vi "Main.vi"() -> ()   [LabVIEW 2017]
doc: "The myRIO Project template acquires acceleration data from the onboard accelerometer and displays the changes of acceleration values in a waveform chart."
uses:
  <vilib>/myRIO/Instrument Drivers/Onboard IO/DIO/typedefs/DIO Reference.ctl
  <vilib>/myRIO/Common/Instrument Driver Framework/Utilities/typedefs/myRIO Generic Hardware Reference.ctl
  <vilib>/myRIO/Common/Instrument Driver Framework/Utilities/typedefs/Hardware Version Enum.ctl
  <vilib>/myRIO/Common/Instrument Driver Framework/Utilities/typedefs/myRIO v1.0 Reference.ctl
  <vilib>/myRIO/Common/Instrument Driver Framework/Utilities/typedefs/Generic FPGA Reference.ctl
  <vilib>/myRIO/Common/Instrument Driver Framework/myRIO v1.0/DIO/typedefs/DIO Channels List.ctl
  <vilib>/myRIO/Common/Instrument Driver Framework/myRIO v1.0/DIO/typedefs/DIO Channels Enum.ctl
  <vilib>/userdefined/High Color/nirio_resource_hc.ctl
  <vilib>/myRIO/Instrument Drivers/Onboard Devices/Accelerometer/typedefs/Accelerometer Reference.ctl
  <vilib>/myRIO/Common/Instrument Driver Framework/myRIO v1.0/Accelerometer/typedefs/Accelerometer Channels List.ctl
  <vilib>/myRIO/Common/Instrument Driver Framework/myRIO v1.0/Accelerometer/typedefs/Accelerometer Channels Enum.ctl
  <vilib>/myRIO/Instrument Drivers/Onboard IO/AI/typedefs/AI Reference.ctl
  <vilib>/myRIO/Common/Instrument Driver Framework/myRIO v1.0/AI/typedefs/AI Channels List.ctl
  <vilib>/myRIO/Common/Instrument Driver Framework/myRIO v1.0/AI/typedefs/AI Channels Enum.ctl
  <vilib>/myRIO/Common/Instrument Driver Framework/Utilities/typedefs/Analog Scaling Constants List.ctl
  <vilib>/myRIO/Common/Instrument Driver Framework/Utilities/typedefs/Analog Scaling Constants.ctl
  <vilib>/myRIO/Common/Instrument Driver Framework/Utilities/vis/Is FPGA Ref Available.vi
  <vilib>/myRIO/Common/Instrument Driver Framework/myRIO v1.0/DIO/vis/myRIO v1.1 Open DIO.vi
  <vilib>/myRIO/Instrument Drivers/Onboard IO/DIO/vis/Write.vi
  <vilib>/myRIO/Common/Instrument Driver Framework/myRIO v1.0/AI/vis/myRIO v1.1 Open AI.vi
  <vilib>/myRIO/Instrument Drivers/Onboard IO/AI/vis/Read.vi
  <vilib>/myRIO/Instrument Drivers/Onboard IO/DIO/vis/Read.vi
  <vilib>/myRIO/Common/Instrument Driver Framework/myRIO v1.0/Accelerometer/vis/myRIO v1.1 Open Accelerometer.vi
  <vilib>/myRIO/Instrument Drivers/Onboard Devices/Accelerometer/vis/Read.vi
  <vilib>/myRIO/Common/Instrument Driver Framework/Utilities/vis/Validate Channels.vi
  <vilib>/myRIO/Common/Instrument Driver Framework/myRIO v1.0/DIO/vis/myRIO v1.0 Reserve DIO.vi
  <vilib>/myRIO/Common/Instrument Driver Framework/myRIO v1.0/AI/vis/myRIO v1.0 Reserve AI.vi
  <vilib>/myRIO/Common/Instrument Driver Framework/myRIO v1.0/Accelerometer/vis/myRIO v1.0 Reserve Accelerometer.vi
  <vilib>/myRIO/Common/Instrument Driver Framework/myRIO v1.0/UART/vis/myRIO v1.0 Close UART.vi
  <vilib>/myRIO/Common/Instrument Driver Framework/myRIO v1.0/Resource Manager/vis/myRIO v1.0 Reserve Channel List.vi
  <vilib>/myRIO/Common/Instrument Driver Framework/myRIO v1.0/DIO/vis/myRIO v1.0 Build MUX Configuration DIO.vi
  <vilib>/myRIO/Common/Instrument Driver Framework/myRIO v1.0/AI/vis/myRIO v1.0 Build MUX Configuration AI.vi
  <vilib>/myRIO/Common/Instrument Driver Framework/myRIO v1.0/Accelerometer/vis/myRIO v1.0 Build MUX Configuration Accelerometer.vi
  <vilib>/myRIO/Common/Instrument Driver Framework/myRIO v1.0/Resource Manager/vis/myRIO v1.0 Reserve Channel.vi
  <vilib>/myRIO/Common/Instrument Driver Framework/myRIO v1.0/Resource Manager/vis/myRIO v1.0 Unreserve Channel.vi
  <vilib>/myRIO/Common/Instrument Driver Framework/myRIO v1.0/Resource Manager/vis/myRIO v1.0 Create Configuration List.vi
  <vilib>/myRIO/Common/Instrument Driver Framework/myRIO v1.0/Resource Manager/vis/myRIO v1.0 Build Mutex Name.vi
  globals.vi
  <vilib>/Utility/VariantDataType/GetNumericInfo.vi
  <vilib>/Utility/error.llb/Error Cluster From Error Code.vi
  <vilib>/myRIO/Common/Instrument Driver Framework/myRIO v1.0/myRIO v1.1 Open.vi
  <vilib>/myRIO/Common/Instrument Driver Framework/myRIO v1.0/Accelerometer/vis/myRIO v1.0 Get Scaling Constant Accelerometer.vi
  <vilib>/myRIO/Common/Instrument Driver Framework/Utilities/vis/IO Manager.vi
  <vilib>/myRIO/Common/Instrument Driver Framework/Utilities/vis/Configuration Manager.vi
  <vilib>/myRIO/Common/Instrument Driver Framework/myRIO v1.0/myRIO v1.0 Close.vi
  <vilib>/myRIO/Common/Instrument Driver Framework/myRIO v1.0/Accelerometer/vis/myRIO v1.0 Read Accelerometer.vi
  <vilib>/myRIO/Common/Instrument Driver Framework/myRIO v1.0/Resource Manager/vis/myRIO v1.0 Configure IO.vi
  <vilib>/myRIO/Common/Instrument Driver Framework/myRIO v1.0/DIO/vis/myRIO v1.0 Read DIO.vi
  <vilib>/myRIO/Common/Instrument Driver Framework/myRIO v1.0/AI/vis/myRIO v1.0 Get Scaling Constants AI.vi
  <vilib>/myRIO/Common/Instrument Driver Framework/myRIO v1.0/AI/vis/myRIO v1.0 Read AI.vi
  <vilib>/myRIO/Common/Instrument Driver Framework/myRIO v1.0/DIO/vis/myRIO v1.0 Write DIO.vi
  <vilib>/myRIO/Common/Instrument Driver Framework/Utilities/vis/FPGA Ref Manager.vi
  <vilib>/myRIO/Common/Instrument Driver Framework/myRIO v1.0/myRIO v1.0 Reset FPGA.vi
  <vilib>/myRIO/Common/Instrument Driver Framework/myRIO v1.0/IRQ/vis/myRIO v1.0 IRQ Info FGV.vi
  <vilib>/myRIO/Common/Instrument Driver Framework/myRIO v1.0/IRQ/vis/myRIO v1.0 Timer IRQ Info FGV.vi
  <vilib>/myRIO/Common/Instrument Driver Framework/myRIO v1.0/IRQ/vis/myRIO v1.0 ISR Agent.vi
  <vilib>/myRIO/Express VI/Onboard Devices/Accelerometer/Accelerometer Express VI.xnode
  <vilib>/myRIO/Instrument Drivers/Onboard Devices/Accelerometer/vis/myRIO Accelerometer Open.xnode
  <vilib>/myRIO/Express VI/Onboard Devices/Button/Button Express VI.xnode
  <vilib>/myRIO/Instrument Drivers/Onboard IO/DIO/vis/myRIO DIO Open.xnode
  <vilib>/myRIO/Express VI/Onboard IO/AI/AI Express VI.xnode
  <vilib>/myRIO/Instrument Drivers/Onboard IO/AI/vis/myRIO AI Open.xnode
  <vilib>/myRIO/Express VI/Onboard Devices/LED/LED Express VI.xnode
  <vilib>/myRIO/Instrument Drivers/Utilities/Utilities.lvlib
  <vilib>/myRIO/Instrument Drivers/Onboard IO/AI/AI.lvlib
  <vilib>/myRIO/Instrument Drivers/Onboard IO/DIO/DIO.lvlib
  <vilib>/myRIO/Instrument Drivers/Onboard Devices/Accelerometer/Accelerometer.lvlib
panel:
  out "theft text":string
  out "Anti-Theft System Active":bool
  out "Local Request From Main":bool
  out "flag4":bool
  out "flag3":bool
  out "flag2":bool
  out "flag1":bool
  out "Count Down":dbl
  out "distance":dbl
  in  "setPos":bool
  out "y":dbl
  out "z":dbl
  out "x":dbl
  in  "correctPass":bool
  out "Main Controller Status":string
  out "String 2":string
  in  "Button":bool
  out "Slide 2":u8(slide) scale=0.0..100.0
  out "String":string
  out "Status":dbl
  out "buff":dbl
  in  "Main Controller IP":string
  out "Thermometer 2":dbl(slide) scale=10.0..35.0
  out "temp":dbl
  out "Slide":u8(slide) scale=0.0..100.0
  # "- If the local controller is disconected from the main controller, local cooling (Arming) is activated\n\n- Local Controller and Main controller start in the local state.\n\n- To terminate local control, hold the local controller button on the MyRio Device. A password will be sent to main controller.\n\n- To enter local cooling manually, hold the local controller button after a request has been given by the main controller to enter local cooling.\n\n- On the main controller, hold down the \"Enable Local Cooling\" Button to toggle the state. When  the state is true, the local controller button can be pressed to activate local cooling"
  # "- When the Anti-Theft system is active, moving the device will trigger the Detonation sequence. 2 different thresholds can be set in the block diagram. The distance of the movement, and the duration of the movement. The duration is there to prevent the  device being triggered by quick vibrations.\n\n- After being triggered, it will countdown from 60 seconds. This can only be deactivated from the main controller with a password.\n\n- After detonation, it will be stuck in an Inert state and can no longer be used."
  # "Statuses\n\n0 - Waiting\n1 - Main Cooling\n2 - Local Cooling\n3 - Detonation\n4 - Detonated"
  # "Detonation Alert"
  # "Nuclear Rod"
  # "Both Need to be activated to Start Local Control"
  # "Local Controller Button"
  # "The local controller and main controller will always attempt to connect to eachother when possible. Make sure the IPs at both ends are correct."
  # "(Hold For 2 Seconds)"
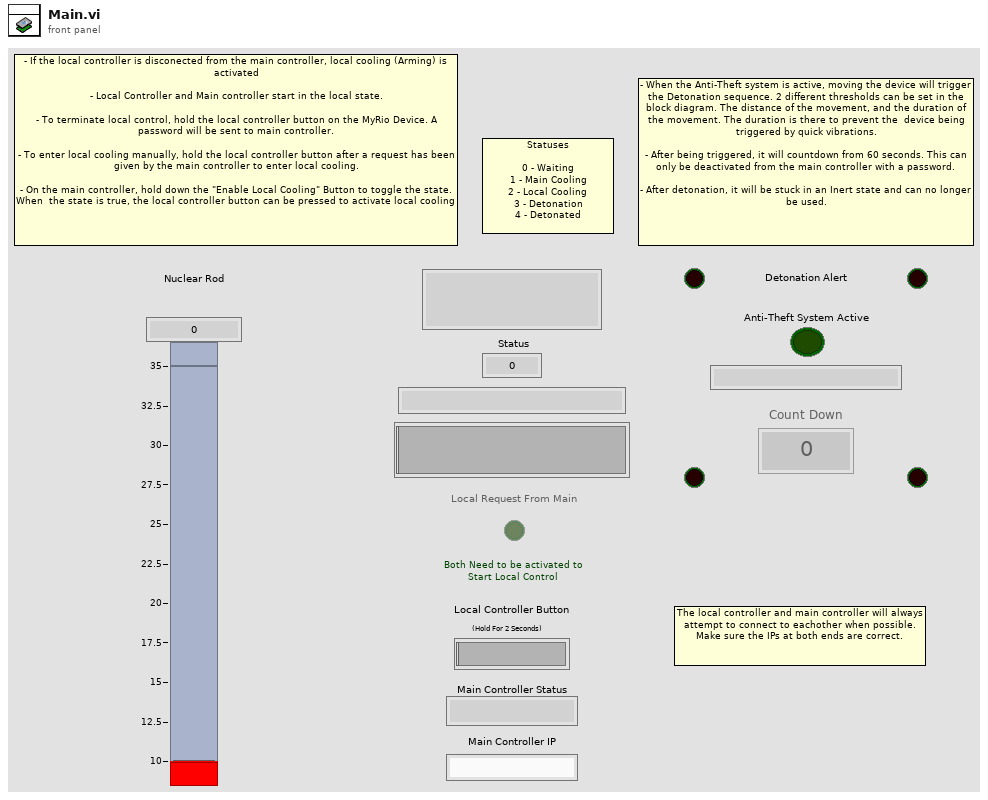
[diagram p1: front panel]
types:
  T1 = typedef "DIO.lvlib/DIO Reference.ctl" = cluster{"myRIO Reference":T2, "DIO Channels List":T6}
  T2 = typedef "myRIO Generic Hardware Reference.ctl" = cluster{"myRIO Model":T3, "myRIO Hardware Reference":T4}
  T3 = typedef "Hardware Version Enum.ctl" = enum16{"Unknown", "myRIO-1900", "myRIO-1950", "roboRIO", "NI ELVIS RIO CM"}
  T4 = typedef "myRIO v1.0 Reference.ctl" = cluster{"Generic FPGA Reference":T5, "Allow multiple opens":bool}
  T5 = typedef "Generic FPGA Reference.ctl" = refnum<k20>
  T6 = typedef "DIO Channels List.ctl" = T7[]
  T7 = typedef "DIO Channels Enum.ctl" = enum16{"Not Connected", "C/DIO0", "C/DIO1", "C/DIO2", "C/DIO3", "C/DIO4", "C/DIO5", "C/DIO6", "C/DIO7", "A/DIO0", "A/DIO1", "A/DIO2", "A/DIO3", "A/DIO4", "A/DIO5", "A/DIO6", "A/DIO7", "A/DIO8", "A/DIO9", "A/DIO10", "A/DIO11", "A/DIO12", "A/DIO13", "A/DIO14", "A/DIO15", "B/DIO0", "B/DIO1", "B/DIO2", "B/DIO3", "B/DIO4", "B/DIO5", "B/DIO6", "B/DIO7", "B/DIO8", "B/DIO9", "B/DIO10", "B/DIO11", "B/DIO12", "B/DIO13", "B/DIO14", "B/DIO15", "LED0", "LED1", "LED2", "LED3", "Button0", "DIO/DIO0", "DIO/DIO1", "DIO/DIO2", "DIO/DIO3", "DIO/DIO4", "DIO/DIO5", "DIO/DIO6", "DIO/DIO7", "DIO/DIO8", "DIO/DIO9", "SPI/CS0", "SPI/CS1", "SPI/CS2", "SPI/CS3", "LED RADIO (Green)", "LED RADIO (Red)", "LED COMM (Green)", "LED COMM (Red)", "LED MODE (Green)", "LED MODE (Red)"}
  T8 = typedef "nirio_resource_hc.ctl" = tag
  T9 = typedef "Accelerometer.lvlib/Accelerometer Reference.ctl" = cluster{"myRIO Reference":T2, "Accelerometer Channels List":T10, "LSB Weight":dbl}
  T10 = typedef "Accelerometer Channels List.ctl" = T11[]
  T11 = typedef "Accelerometer Channels Enum.ctl" = enum16{"Not Connected", "X-Axis", "Y-Axis", "Z-Axis"}
  T12 = typedef "AI.lvlib/AI Reference.ctl" = cluster{"myRIO Reference":T2, "AI Channels List":T13, "AI Scaling Constants List":T15}
  T13 = typedef "AI Channels List.ctl" = T14[]
  T14 = typedef "AI Channels Enum.ctl" = enum16{"Not Connected", "AudioIn/Left", "AudioIn/Right", "C/AI0", "C/AI1", "A/AI0", "A/AI1", "A/AI2", "A/AI3", "B/AI0", "B/AI1", "B/AI2", "B/AI3", "AI/AI0", "AI/AI1", "AI/AI2", "AI/AI3"}
  T15 = typedef "Analog Scaling Constants List.ctl" = T16[]
  T16 = typedef "Analog Scaling Constants.ctl" = cluster{"LSB Weight (Volts)":dbl, "Offset (Volts)":dbl, "Signed?":bool}
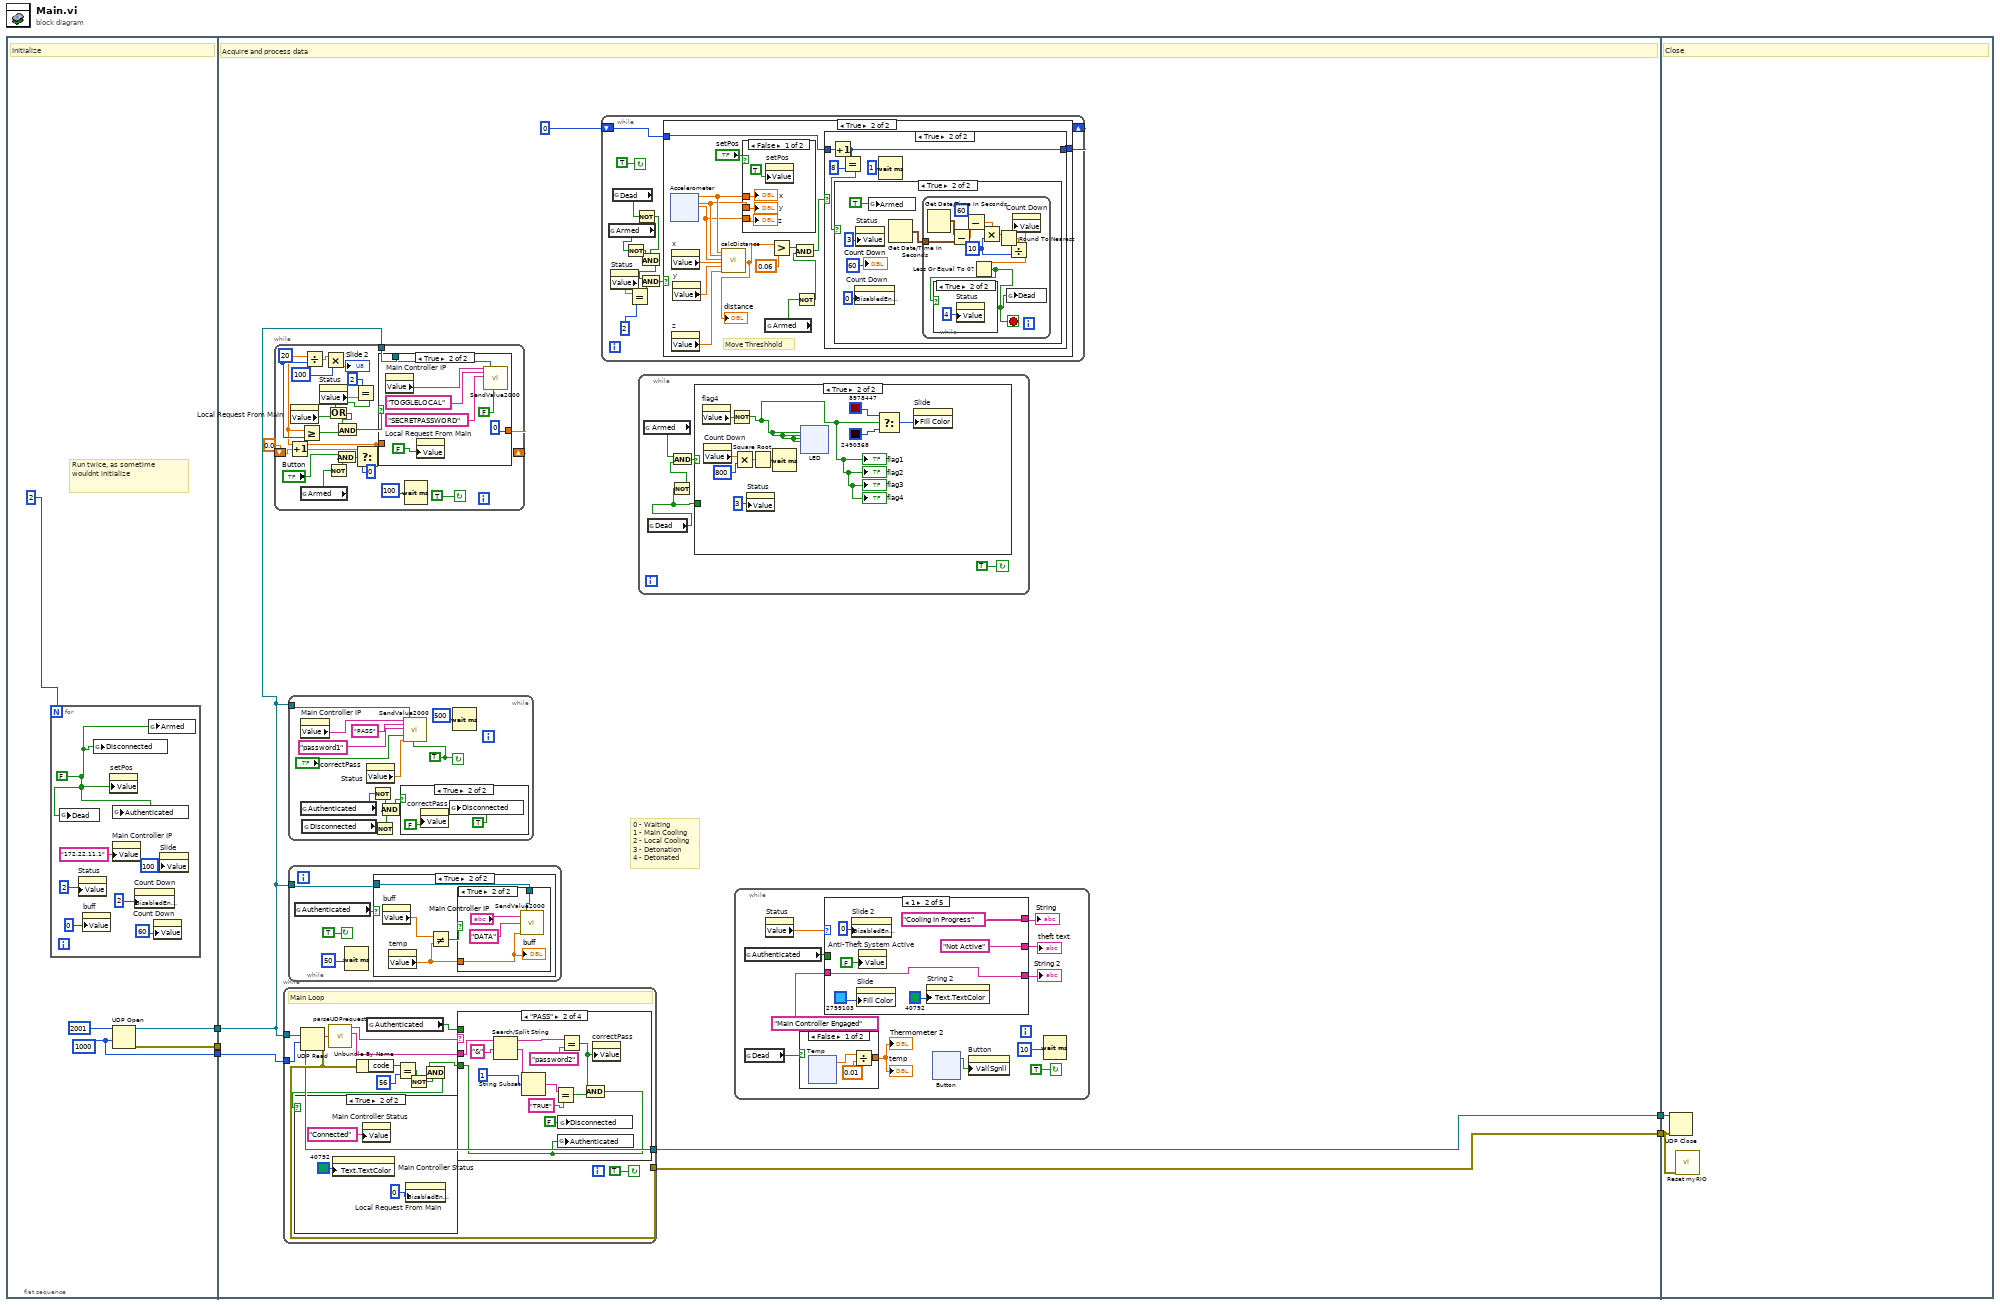
[diagram p0: block diagram]
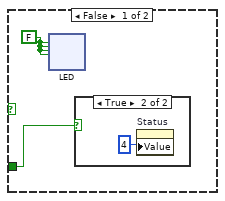
[diagram p2: hidden frame]
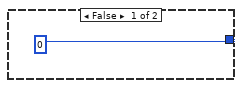
[diagram p4: hidden frame]
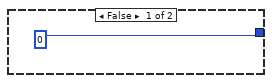
[diagram p5: hidden frame]
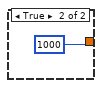
[diagram p13: hidden frame]
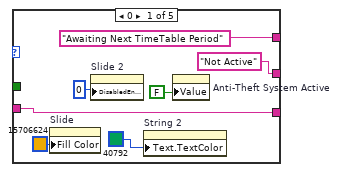
[diagram p14: hidden frame]
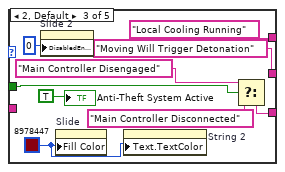
[diagram p15: hidden frame]
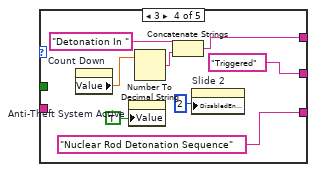
[diagram p16: hidden frame]
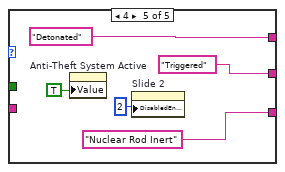
[diagram p17: hidden frame]
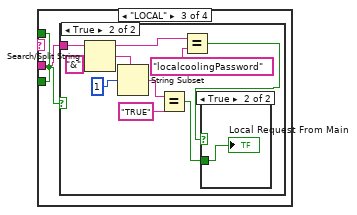
[diagram p19: hidden frame]
diagram:
  n1 = flat-sequence {
    tunnel: [w9] -> w5
    tunnel: [w8] -> w4
    tunnel: [w7] -> w3
    tunnel: w5 -> [w19]
    tunnel: w4 -> [_]
    tunnel: w3 -> [w23]
    tunnel: [w22] -> w2
    tunnel: [w21] -> w1
    tunnel: w2 -> [w463]
    tunnel: w1 -> [w464]
    frame #0 {
      w7 = 1000
      # "Run twice, as sometime wouldnt initialize"
      # "Initialize"
      n2 = for {
        N: 2 -> [_]
        w11 = FALSE
        n3 = global write "globals.vi" "Dead"(w11) -> ()
        n4 = property on="Status" class="DigNum (strict)"("Value"=2) -> ()  [unwired: 2 in, 2 out]
        n5 = property on="buff" class="DigNum (strict)"("Value"=0) -> ()  [unwired: 2 in, 2 out]
        n6 = global write "globals.vi" "Disconnected"(w11) -> ()
        n7 = property on="setPos" class="Bool (strict)"("Value"=w11) -> ()  [unwired: 2 in, 2 out]
        n8 = global write "globals.vi" "Authenticated"(w11) -> ()
        n9 = property on="Main Controller IP" class="Str"("Value"="172.22.11.1") -> ()  [unwired: 2 in, 2 out]
        n10 = property on="Count Down" class="DigNum (strict)"("DisabledEnum"=2) -> ()  [unwired: 2 in, 2 out]
        n11 = global write "globals.vi" "Armed"(w11) -> ()
        n12 = property on="Count Down" class="DigNum (strict)"("Value"=60) -> ()  [unwired: 2 in, 2 out]
        n13 = property on="Slide" class="Slide (strict)"("Value"=100) -> ()  [unwired: 2 in, 2 out]
      }
      n14 = UDP Open(9:w7, 11:u16 2001 ("port")) -> (port=w9:refnum<k16>, 0:w8:errorcluster)  [unwired: 3 in, 1 out]
    }
    frame #1 {
      # "0 - Waiting\n1 - Main Cooling\n2 - Local Cooling\n3 - Detonation\n4 - Detonated"
      # "Acquire and process data"
      n15 = while {
        shift-right: [w226] -> _
        shift-left: 0.0 ("f") -> [w233]
        tunnel: w19 -> [w223]
        stop <- TRUE continue-if-true
        w229 = 20
        n16 = Increment(x=w233) -> (x+1=w228:dbl)
        n17 = property on="Local Request From Main" class="Bool (strict)"() -> ("Value"=w214:bool)  [unwired: 2 in, 2 out]
        n18 = global read "globals.vi" "Armed"() -> (w211:bool)
        n19 = property on="Status" class="DigNum (strict)"() -> ("Value"=w217:dbl)  [unwired: 2 in, 2 out]
        n20 = Not(x=w211) -> (.not. x?=w212:bool)
        n21 = And(x="Button", y=w212) -> (x .and. y?=w221:bool)
        n22 = Equal?(x=2, y=w217) -> (x = y?=w213:bool)
        n23 = Or(x=w213, y=w214) -> (x .or. y?=w215:bool)
        n24 = Select(t=w228, s=w221, f=0) -> (s? t:f=w218:dbl)
        n25 = Greater Or Equal?(x=w218, y=w229) -> (x >= y?=w220:bool)
        n26 = Divide(x=w218, y=w229) -> (x/y=w231:dbl)
        n27 = Multiply(x=w231, y=100) -> (x*y=→"Slide 2":dbl)
        n28 = And(x=w215, y=w220) -> (x .and. y?=w219:bool)
        n29 = case shown="True" w219 {
          tunnel: [w234 0] -> w226
          tunnel: w218 -> [w234 _]
          tunnel: w223 -> [_ w240]
          frame False {
          }
          frame True {
            n30 = property on="Main Controller IP" class="Str"() -> ("Value"=w238:string)  [unwired: 2 in, 2 out]
            n31 = property on="Local Request From Main" class="Bool (strict)"("Value"=FALSE) -> ()  [unwired: 2 in, 2 out]
            n32 = call "SendValue2000.vi"("ip"=w238, "command"="TOGGLELOCAL", "Stringvalue"="SECRETPASSWORD", "connection ID"=w240, "Send Bool"=FALSE) -> ()  [unwired: 15 in]
          }
        }
        n33 = Wait (ms)(milliseconds to wait=100) -> ()  [unwired: 1 out]
      }
      n34 = while {
        tunnel: w23 -> [w402]
        tunnel: [w398] -> w22
        tunnel: w19 -> [w397]
        tunnel: [w397] -> w21
        tunnel: [w397] -> _
        stop <- TRUE continue-if-true
        # "Main Loop"
        n35 = UDP Read(connection ID=w397, timeout ms (25000)=w402) -> (data out=w399:string, error out=w398:errorcluster)  [unwired: 2 in, 3 out]
        n36 = call "parseUDPrequest.vi"("data"=w399) -> ("value"=w400:string, "command"=w401:string)  [unwired: 9 in]
        n37 = Unbundle By Name(w398) -> ("code"=w403:i32)
        n38 = global read "globals.vi" "Authenticated"() -> (w392:bool)
        n39 = Equal?(x=w403, y=56) -> (x = y?=w396:bool)
        n40 = Not(x=w396) -> (.not. x?=w395:bool)
        n41 = case shown="\"PASS\"" w401 {
          tunnel: w400 -> [_ w414 w419 w439]
          tunnel: w392 -> [w406 _ w420 w438]
          tunnel: [w406 w407 w420 w438] -> w394
          frame "False", Default {
          }
          frame "PASS" {
            n42 = Search/Split String(string=w414, search string/char (-)="&") -> (substring before match=w413:string, match + rest of string=w417:string)  [unwired: 1 in, 1 out]
            n43 = String Subset(string=w417, offset (0)=1) -> (substring=w411:string)  [unwired: 1 in]
            n44 = Equal?(x=w411, y="TRUE") -> (x = y?=w410:bool)
            n45 = global write "globals.vi" "Disconnected"(FALSE) -> ()
            n46 = Equal?(x=w413, y="password2") -> (x = y?=w409:bool)
            n47 = And(x=w409, y=w410) -> (x .and. y?=w407:bool)
            n48 = global write "globals.vi" "Authenticated"(w407) -> ()
            n49 = property on="correctPass" class="Bool (strict)"("Value"=w409) -> ()  [unwired: 2 in, 2 out]
          }
          frame "LOCAL" {
            n50 = case shown="True" w420 {
              tunnel: w419 -> [_ w423]
              frame False {
              }
              frame True {
                n51 = Search/Split String(string=w423, search string/char (-)="&") -> (substring before match=w426:string, match + rest of string=w425:string)  [unwired: 1 in, 1 out]
                n52 = String Subset(string=w425, offset (0)=1) -> (substring=w430:string)  [unwired: 1 in]
                n53 = Equal?(x=w430, y="TRUE") -> (x = y?=w421:bool)
                n54 = Equal?(x=w426, y="localcoolingPassword") -> (x = y?=w422:bool)
                n55 = case shown="True" w422 {
                  tunnel: w421 -> [_ w431]
                  frame False {
                  }
                  frame True {
                    "Local Request From Main" <- w431
                  }
                }
              }
            }
          }
          frame "DATA" {
            n56 = global read "globals.vi" "Armed"() -> (w432:bool)
            n57 = Not(x=w432) -> (.not. x?=w435:bool)
            n58 = global read "globals.vi" "Dead"() -> (w433:bool)
            n59 = Not(x=w433) -> (.not. x?=w434:bool)
            n60 = And(x=w434, y=w435) -> (x .and. y?=w436:bool)
            n61 = And(x=w436, y=w438) -> (x .and. y?=w437:bool)
            n62 = case shown="True" w437 {
              tunnel: w439 -> [_ w446]
              frame False {
              }
              frame True {
                n63 = Search/Split String(string=w446, search string/char (-)="&") -> (substring before match=w444:string, match + rest of string=w442:string)  [unwired: 1 in, 1 out]
                n64 = String Subset(string=w442, offset (0)=1) -> (substring=w441:string)  [unwired: 1 in]
                n65 = Decimal String To Number(string=w441) -> (number=→"Status":i32)  [unwired: 2 in, 1 out]
                n66 = Decimal String To Number(string=w444) -> (number=→"Slide":i32)  [unwired: 2 in, 1 out]
              }
            }
          }
        }
        n67 = And(x=w394, y=w395) -> (x .and. y?=w393:bool)
        n68 = case shown="True" w393 {
          frame False {
            n69 = property on="Main Controller Status" class="Str"("Text.TextColor"=u32 8978447) -> ()  [unwired: 2 in, 2 out]
            n70 = global write "globals.vi" "Authenticated"(FALSE) -> ()
            n71 = property on="Slide" class="Slide (strict)"("Value"=100) -> ()  [unwired: 2 in, 2 out]
            n72 = property on="Local Request From Main" class="Bool (strict)"("Value"=FALSE) -> ()  [unwired: 2 in, 2 out]
            n73 = global read "globals.vi" "Armed"() -> (w448:bool)
            n74 = global read "globals.vi" "Dead"() -> (w450:bool)
            n75 = property on="Local Request From Main" class="Bool (strict)"("DisabledEnum"=2) -> ()  [unwired: 2 in, 2 out]
            n76 = Not(x=w450) -> (.not. x?=w455:bool)
            n77 = And(x=w455, y=w448) -> (x .and. y?=w454:bool)
            n78 = case shown="False" w454 {
              frame False {
                n79 = property on="Status" class="DigNum (strict)"("Value"=2) -> ()  [unwired: 2 in, 2 out]
              }
              frame True {
                n80 = property on="Status" class="DigNum (strict)"("Value"=3) -> ()  [unwired: 2 in, 2 out]
              }
            }
            "Main Controller Status" <- "Disconnected"
          }
          frame True {
            n81 = property on="Main Controller Status" class="Str"("Text.TextColor"=u32 40792) -> ()  [unwired: 2 in, 2 out]
            n82 = property on="Main Controller Status" class="Str"("Value"="Connected") -> ()  [unwired: 2 in, 2 out]
            n83 = property on="Local Request From Main" class="Bool (strict)"("DisabledEnum"=0) -> ()  [unwired: 2 in, 2 out]
          }
        }
      }
      n84 = while {
        tunnel: w19 -> [w253]
        stop <- w245 continue-if-true
        w245 = TRUE
        n85 = global read "globals.vi" "Authenticated"() -> (w242:bool)
        n86 = property on="Main Controller IP" class="Str"() -> ("Value"=w254:string)  [unwired: 2 in, 2 out]
        n87 = global read "globals.vi" "Disconnected"() -> (w243:bool)
        n88 = property on="Status" class="DigNum (strict)"() -> ("Value"=w244:dbl)  [unwired: 2 in, 2 out]
        n89 = Not(x=w242) -> (.not. x?=w247:bool)
        n90 = Not(x=w243) -> (.not. x?=w248:bool)
        n91 = And(x=w247, y=w248) -> (x .and. y?=w246:bool)
        n92 = case shown="True" w246 {
          frame False {
          }
          frame True {
            n93 = property on="correctPass" class="Bool (strict)"("Value"=FALSE) -> ()  [unwired: 2 in, 2 out]
            n94 = global write "globals.vi" "Disconnected"(TRUE) -> ()
          }
        }
        n95 = call "SendValue2000.vi"("ip"=w254, "command"="PASS", "Stringvalue"="password1", "Boolean"="correctPass", "value"=w244, "connection ID"=w253, "Send Bool"=w245) -> ()  [unwired: 13 in]
        n96 = Wait (ms)(milliseconds to wait=500) -> ()  [unwired: 1 out]
      }
      n97 = while {
        tunnel: w19 -> [w259]
        stop <- TRUE continue-if-true
        n98 = global read "globals.vi" "Authenticated"() -> (w257:bool)
        n99 = Wait (ms)(milliseconds to wait=50) -> ()  [unwired: 1 out]
        n100 = case shown="True" w257 {
          tunnel: w259 -> [_ w264]
          frame False {
          }
          frame True {
            n101 = property on="buff" class="DigNum (strict)"() -> ("Value"=w263:dbl)  [unwired: 2 in, 2 out]
            n102 = property on="temp" class="DigNum (strict)"() -> ("Value"=w262:dbl)  [unwired: 2 in, 2 out]
            n103 = Not Equal?(x=w263, y=w262) -> (x != y?=w261:bool)
            n104 = case shown="True" w261 {
              tunnel: w264 -> [_ w267]
              tunnel: w262 -> [_ w265]
              frame False {
              }
              frame True {
                n105 = call "SendValue2000.vi"("ip"="Main Controller IP", "command"="DATA", "value"=w265, "connection ID"=w267) -> ()  [unwired: 16 in]
                "buff" <- w265
              }
            }
          }
        }
      }
      n106 = while {
        shift-right: [w125] -> _
        shift-left: 0 -> [w127]
        stop <- TRUE continue-if-true
        n107 = global read "globals.vi" "Armed"() -> (w118:bool)
        n108 = property on="Status" class="DigNum (strict)"() -> ("Value"=w128:dbl)  [unwired: 2 in, 2 out]
        n109 = global read "globals.vi" "Dead"() -> (w119:bool)
        n110 = Not(x=w118) -> (.not. x?=w121:bool)
        n111 = Equal?(x=w128, y=2) -> (x = y?=w124:bool)
        n112 = Not(x=w119) -> (.not. x?=w122:bool)
        n113 = And(x=w122, y=w121) -> (x .and. y?=w120:bool)
        n114 = And(x=w120, y=w124) -> (x .and. y?=w123:bool)
        n115 = case shown="True" w123 {
          tunnel: w127 -> [_ w134]
          tunnel: [0 w133] -> w125
          frame False {
          }
          frame True {
            # "Move Threshhold"
            n116 = xnode "Accelerometer"() -> ("X-Axis"=w144:dbl, "Y-Axis"=w143:dbl, "Z-Axis"=w142:dbl)  [unwired: 1 in, 1 out]
            n117 = property on="x" class="DigNum (strict)"() -> ("Value"=w141:dbl)  [unwired: 2 in, 2 out]
            n118 = property on="z" class="DigNum (strict)"() -> ("Value"=w139:dbl)  [unwired: 2 in, 2 out]
            n119 = property on="y" class="DigNum (strict)"() -> ("Value"=w140:dbl)  [unwired: 2 in, 2 out]
            n120 = call "calcDistance.vi"("currentPos x"=w144, "currentPos y"=w143, "currentPos z"=w142, "savedPos x"=w141, "savedPos y"=w140, "savedPos z"=w139) -> ("Numeric"=w137:dbl)  [unwired: 13 in]
            "distance" <- w137
            n121 = case shown="False" "setPos" {
              tunnel: w144 -> [w171 _]
              tunnel: w143 -> [w170 _]
              tunnel: w142 -> [w169 _]
              frame False {
                n122 = property on="setPos" class="Bool (strict)"("Value"=TRUE) -> ()  [unwired: 2 in, 2 out]
                "x" <- w171
                "y" <- w170
                "z" <- w169
              }
              frame True {
              }
            }
            n123 = global read "globals.vi" "Armed"() -> (w131:bool)
            n124 = Greater?(x=w137, y=0.06) -> (0:w136:bool)
            n125 = Not(x=w131) -> (.not. x?=w135:bool)
            n126 = And(x=w136, y=w135) -> (x .and. y?=w132:bool)
            n127 = case shown="True" w132 {
              tunnel: w134 -> [_ w149]
              tunnel: [0 w148] -> w133
              frame False {
              }
              frame True {
                n128 = Increment(x=w149) -> (x+1=w148:i32)
                n129 = Equal?(x=w148, y=8) -> (x = y?=w150:bool)
                n130 = case shown="True" w150 {
                  frame False {
                  }
                  frame True {
                    n131 = property on="Count Down" class="DigNum (strict)"("DisabledEnum"=0) -> ()  [unwired: 2 in, 2 out]
                    n132 = property on="Status" class="DigNum (strict)"("Value"=3) -> ()  [unwired: 2 in, 2 out]
                    n133 = global write "globals.vi" "Armed"(TRUE) -> ()
                    n134 = Get Date/Time In Seconds() -> (seconds since 1Jan1904=w153:timestamp)
                    n135 = while {
                      tunnel: w153 -> [w158]
                      stop <- w157 stop-if-true
                      w160 = 10
                      n136 = Get Date/Time In Seconds() -> (seconds since 1Jan1904=w161:timestamp)
                      n137 = Subtract(x=w161, y=w158) -> (x-y=w162:dbl)
                      n138 = Subtract(x=60, y=w162) -> (x-y=w163:dbl)
                      n139 = Multiply(x=w163, y=w160) -> (x*y=w164:dbl)
                      n140 = Round To Nearest(number=w164) -> (nearest integer value=w165:dbl)
                      n141 = Divide(x=w165, y=w160) -> (x/y=w166:dbl)
                      n142 = Less Or Equal To 0?(x=w166) -> (x <= 0?=w157:bool)
                      n143 = case shown="True" w157 {
                        frame False {
                        }
                        frame True {
                          n144 = property on="Status" class="DigNum (strict)"("Value"=4) -> ()  [unwired: 2 in, 2 out]
                        }
                      }
                      n145 = global write "globals.vi" "Dead"(w157) -> ()
                      n146 = property on="Count Down" class="DigNum (strict)"("Value"=w166) -> ()  [unwired: 2 in, 2 out]
                    }
                    "Count Down" <- 60
                  }
                }
                n147 = Wait (ms)(milliseconds to wait=1) -> ()  [unwired: 1 out]
              }
            }
          }
        }
      }
      n148 = while {
        stop <- TRUE continue-if-true
        n149 = global read "globals.vi" "Armed"() -> (w24:bool)
        n150 = global read "globals.vi" "Dead"() -> (w25:bool)
        n151 = Not(x=w25) -> (.not. x?=w26:bool)
        n152 = And(x=w24, y=w26) -> (x .and. y?=w27:bool)
        n153 = case shown="True" w27 {
          tunnel: w25 -> [w29 _]
          frame False {
            w30 = FALSE
            n154 = xnode "LED"("LED0"=w30, "LED1"=w30, "LED2"=w30, "LED3"=w30) -> ()  [unwired: 1 in, 1 out]
            n155 = case shown="True" w29 {
              frame False {
              }
              frame True {
                n156 = property on="Status" class="DigNum (strict)"("Value"=4) -> ()  [unwired: 2 in, 2 out]
              }
            }
          }
          frame True {
            n157 = property on="flag4" class="Bool (strict)"() -> ("Value"=w70:bool)  [unwired: 2 in, 2 out]
            n158 = property on="Count Down" class="DigNum (strict)"() -> ("Value"=w79:dbl)  [unwired: 2 in, 2 out]
            n159 = Not(x=w70) -> (.not. x?=w71:bool)
            "flag1" <- w71
            "flag2" <- w71
            "flag3" <- w71
            "flag4" <- w71
            n160 = Multiply(x=w79, y=800) -> (x*y=w78:dbl)
            n161 = property on="Status" class="DigNum (strict)"("Value"=3) -> ()  [unwired: 2 in, 2 out]
            n162 = Square Root(x=w78) -> (sqrt(x)=w77:dbl)
            n163 = Wait (ms)(milliseconds to wait=w77) -> ()  [unwired: 1 out]
            n164 = xnode "LED"("LED0"=w71, "LED1"=w71, "LED2"=w71, "LED3"=w71) -> ()  [unwired: 1 in, 1 out]
            n165 = Select(t=u32 8978447, s=w71, f=u32 2490368) -> (s? t:f=w75:u32)
            n166 = property on="Slide" class="Slide (strict)"("Fill Color"=w75) -> ()  [unwired: 2 in, 2 out]
          }
        }
      }
      n167 = while {
        stop <- TRUE continue-if-true
        n168 = global read "globals.vi" "Authenticated"() -> (w269:bool)
        n169 = global read "globals.vi" "Dead"() -> (w270:bool)
        n170 = property on="Status" class="DigNum (strict)"() -> ("Value"=w274:dbl)  [unwired: 2 in, 2 out]
        n171 = case shown="False" w270 {
          tunnel: [w280 1000] -> w273
          frame False {
            n172 = xnode "Temp"() -> ("Temp (A/AI3 (Pin 9))"=w281:dbl)  [unwired: 1 in, 1 out]
            n173 = Divide(x=w281, y=0.01) -> (x/y=w280:dbl)
          }
          frame True {
          }
        }
        "Thermometer 2" <- w273
        "temp" <- w273
        n174 = case shown="1" w274 {
          tunnel: ["Awaiting Next TimeTable Period" "Cooling In Progress" "Local Cooling Running" w384 "Detonated"] -> w277
          tunnel: [w360 w367 w375 "Nuclear Rod Detonation Sequence" "Nuclear Rod Inert"] -> w276
          tunnel: "Main Controller Engaged" -> [w360 w367 _ _ _]
          tunnel: w269 -> [_ _ w372 _ _]
          tunnel: ["Not Active" "Not Active" "Moving Will Trigger Detonation" "Triggered" "Triggered"] -> w271
          frame 0 {
            n175 = property on="Slide" class="Slide (strict)"("Fill Color"=u32 15706624) -> ()  [unwired: 2 in, 2 out]
            n176 = property on="Slide 2" class="Slide (strict)"("DisabledEnum"=0) -> ()  [unwired: 2 in, 2 out]
            n177 = property on="String 2" class="Str"("Text.TextColor"=u32 40792) -> ()  [unwired: 2 in, 2 out]
            n178 = property on="Anti-Theft System Active" class="Bool (strict)"("Value"=FALSE) -> ()  [unwired: 2 in, 2 out]
          }
          frame 1 {
            n179 = property on="Slide 2" class="Slide (strict)"("DisabledEnum"=0) -> ()  [unwired: 2 in, 2 out]
            n180 = property on="Slide" class="Slide (strict)"("Fill Color"=u32 2799103) -> ()  [unwired: 2 in, 2 out]
            n181 = property on="Anti-Theft System Active" class="Bool (strict)"("Value"=FALSE) -> ()  [unwired: 2 in, 2 out]
            n182 = property on="String 2" class="Str"("Text.TextColor"=u32 40792) -> ()  [unwired: 2 in, 2 out]
          }
          frame 2, Default {
            w377 = u32 8978447
            n183 = property on="Slide 2" class="Slide (strict)"("DisabledEnum"=0) -> ()  [unwired: 2 in, 2 out]
            n184 = property on="Slide" class="Slide (strict)"("Fill Color"=w377) -> ()  [unwired: 2 in, 2 out]
            n185 = property on="String 2" class="Str"("Text.TextColor"=w377) -> ()  [unwired: 2 in, 2 out]
            n186 = Select(t="Main Controller Disengaged", s=w372, f="Main Controller Disconnected") -> (s? t:f=w375:string)
            "Anti-Theft System Active" <- TRUE
          }
          frame 3 {
            n187 = property on="Count Down" class="DigNum (strict)"() -> ("Value"=w383:dbl)  [unwired: 2 in, 2 out]
            n188 = property on="Anti-Theft System Active" class="Bool (strict)"("Value"=TRUE) -> ()  [unwired: 2 in, 2 out]
            n189 = Number To Decimal String(number=w383) -> (decimal integer string=w385:string)  [unwired: 1 in]
            n190 = Concatenate Strings("Detonation In ", w385) -> (w384:string)
            n191 = property on="Slide 2" class="Slide (strict)"("DisabledEnum"=2) -> ()  [unwired: 2 in, 2 out]
          }
          frame 4 {
            n192 = property on="Anti-Theft System Active" class="Bool (strict)"("Value"=TRUE) -> ()  [unwired: 2 in, 2 out]
            n193 = property on="Slide 2" class="Slide (strict)"("DisabledEnum"=2) -> ()  [unwired: 2 in, 2 out]
          }
        }
        "String" <- w277
        "String 2" <- w276
        "theft text" <- w271
        n194 = xnode "Button"() -> ("Value"=w278:bool)  [unwired: 1 in, 1 out]
        n195 = property on="Button" class="Bool (strict)"("Val(Sgnl)"=w278) -> ()  [unwired: 2 in, 2 out]
        n196 = Wait (ms)(milliseconds to wait=10) -> ()  [unwired: 1 out]
      }
    }
    frame #2 {
      # "Close"
      n197 = UDP Close(connection ID=w464, 8:w463) -> ()  [unwired: 2 out]
      n198 = call <vilib>:"Reset myRIO.vi"("error in (no error)"=w463) -> ()  [unwired: 10 in, 1 out]
    }
  }
